vi "Abs to Rel Path.vi"(9 "File Path":path, 11 "Base Path":path) -> (1 "Rel Path?":bool, 3 "Path Out":path)   [LabVIEW 2010]
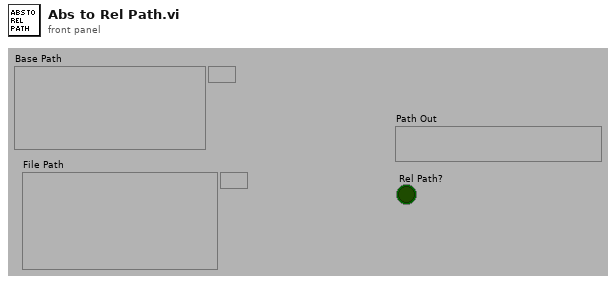
[diagram p1: front panel]
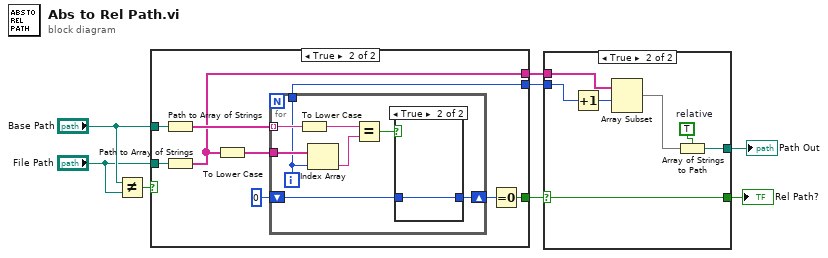
[diagram p0: block diagram]
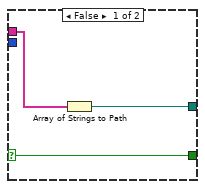
[diagram p2: hidden frame]
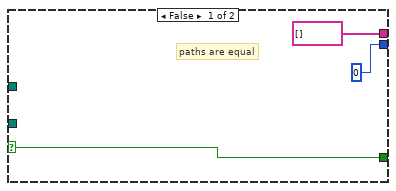
[diagram p3: hidden frame]
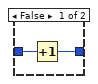
[diagram p4: hidden frame]
diagram:
  n1 = Not Equal?(x="Base Path", y="File Path") -> (x != y?=w6:bool)
  n2 = case shown="True" w6 {
    selector: w6 -> [w11 _]
    tunnel: [w11 w17] -> w5
    tunnel: "Base Path" -> [_ w16]
    tunnel: "File Path" -> [_ w15]
    tunnel: [0 w14] -> w3
    tunnel: [string[] [] ("array of strings") w13] -> w2
    frame False {
      # "paths are equal"
    }
    frame True {
      n3 = Path to Array of Strings(0:w16) -> (2:w20:string[])  [unwired: 1 out]
      n4 = Path to Array of Strings(0:w15) -> (2:w13:string[])  [unwired: 1 out]
      n5 = To Lower Case(string=w13) -> (all lower case string=w12:string[])
      n6 = for {
        tunnel: w20 -> [w26] mode=indexing
        tunnel: w12 -> [w28]
        shift-right: [w25] -> w18
        shift-left: 0 -> [w23]
        tunnel: [w22] -> w14
        i -> [w22]
        n7 = To Lower Case(string=w26) -> (all lower case string=w21:string)
        n8 = Index Array(array=w28, index=w22) -> (element=w27:string)
        n9 = Equal?(x=w21, y=w27) -> (x = y?=w24:bool)
        n10 = case shown="True" w24 {
          tunnel: [w29 w31] -> w25
          tunnel: w23 -> [w30 w31]
          frame False {
            n11 = Increment(x=w30) -> (x+1=w29:i32)
          }
          frame True {
          }
        }
      }
      n12 = Equal To 0?(x=w18) -> (x = 0?=w17:bool)
    }
  }
  n13 = case shown="True" w5 {
    selector: w5 -> [w34 w41]
    tunnel: [w34 w41] -> w4
    tunnel: w3 -> [_ w39]
    tunnel: w2 -> [w33 w40]
    tunnel: [w32 w38] -> w1
    frame False {
      n14 = Array of Strings to Path(0:w33) -> (2:w32:path)  [unwired: 1 in]
    }
    frame True {
      w36 = TRUE  # relative
      n15 = Increment(x=w39) -> (x+1=w35:i32)
      n16 = Array Subset(array=w40, index=w35) -> (w37:string[])  [unwired: 1 in]
      n17 = Array of Strings to Path(0:w37, 1:w36) -> (2:w38:path)
    }
  }
  "Rel Path?" <- w4
  "Path Out" <- w1
